vi "u-blox 5 Series Acquire and Chart GPS Advanced.vi"() -> ()   [LabVIEW 2009]
doc: "This example shows how to utilize the advanced VIs in the u-blox 5 GPS driver. It reads the sentences coming from the GPS device and parses out data for position and dilution of precision."
panel:
  out "Dilution of Precision":dbl
  out "Position":cluster{dbl, dbl}[](graph)
  out "Vertical Dilution of Precision":dbl
  out "Horizontal Dilution of Precision":dbl
  in  "stop":bool
  in  "Reset Before Reading (False)":bool
  in  "VISA resource name":refnum<visa-resource-name>
  # "(c) 2009 National Instruments.  ALL RIGHTS RESERVED."
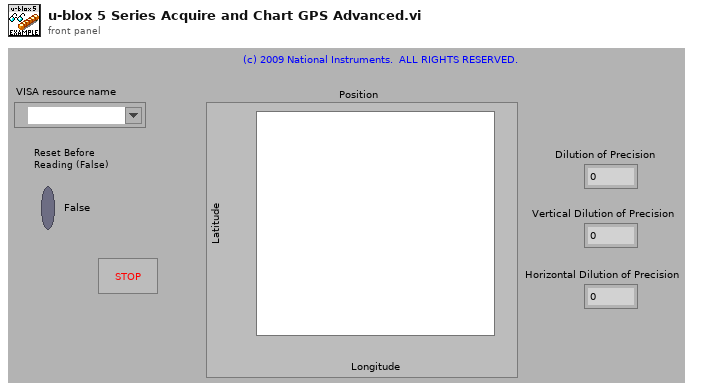
[diagram p1: front panel]
types:
  T1 = cluster{"Dilution of Precision":dbl, "Horizontal Dilution of Precision":dbl, "Vertical Dilution of Precision":dbl}[]
  T2 = cluster{"Timestamp":timestamp, "Latitude":dbl, "Longitude":dbl}[]
  T3 = cluster{"Dilution of Precision":dbl, "Horizontal Dilution of Precision":dbl, "Vertical Dilution of Precision":dbl}
  T4 = cluster{"Timestamp":timestamp, "Latitude":dbl, "Longitude":dbl}
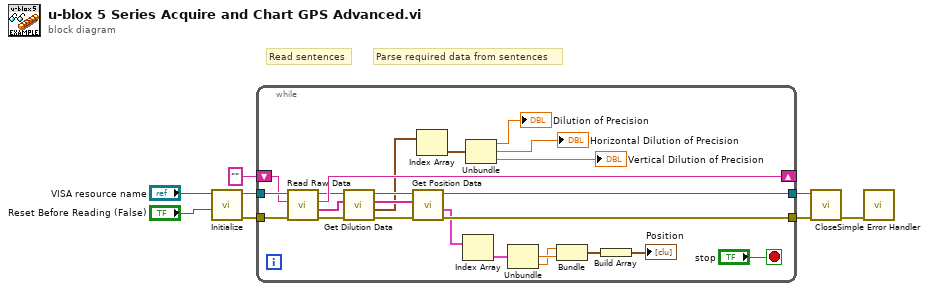
[diagram p0: block diagram]
diagram:
  # "Read sentences"
  # "Parse required data from sentences"
  n1 = call "Initialize.vi"("Reset (False)"="Reset Before Reading (False)", "VISA resource name"="VISA resource name") -> ("error out"=w5:errorcluster, "VISA resource name out"=w6:refnum<visa-resource-name>)  [unwired: 8 in]
  n2 = while {
    tunnel: w6 -> [w32]
    tunnel: w5 -> [w31]
    tunnel: [w22] -> w4
    tunnel: [w21] -> w3
    shift-right: [w29] -> _
    shift-left: "" ("Remaining Partial Sentence") -> [w28]
    stop <- "stop" stop-if-true
    n3 = call "Read Raw Data.vi"("error in (no error)"=w31, "Previous Partial Sentence"=w28, "VISA resource name"=w32) -> ("error out"=w26:errorcluster, "Complete NMEA Sentences"=w17:string[], "Remaining Partial Sentence"=w29:string, "VISA resource name out"=w24:refnum<visa-resource-name>)  [unwired: 5 in]
    n4 = call "Get Dilution Data.vi"("error in (no error)"=w26, "Complete NMEA Sentences"=w17, "VISA resource name"=w24) -> ("error out"=w25:errorcluster, "Dilution Data"=w19:T1, "Complete NMEA Sentences (Copy)"=w20:string[], "VISA resource name out"=w23:refnum<visa-resource-name>)  [unwired: 5 in]
    n5 = call "Get Position Data.vi"("error in (no error)"=w25, "Complete NMEA Sentences"=w20, "VISA resource name"=w23) -> ("error out"=w21:errorcluster, "Position Data"=w18:T2, "VISA resource name out"=w22:refnum<visa-resource-name>)  [unwired: 5 in, 1 out]
    n6 = Index Array(array=w19) -> (element=w16:T3)  [unwired: 1 in]
    n7 = Index Array(array=w18) -> (element=w27:T4)  [unwired: 1 in]
    n8 = Unbundle(w16) -> ("Dilution of Precision"=→"Dilution of Precision":dbl, "Horizontal Dilution of Precision"=→"Horizontal Dilution of Precision":dbl, "Vertical Dilution of Precision"=→"Vertical Dilution of Precision":dbl)
    n9 = Unbundle(w27) -> ("Latitude"=w13:dbl, "Longitude"=w12:dbl)  [unwired: 1 out]
    n10 = Bundle("Longitude"=w12, "Latitude"=w13) -> (w11:cluster{"Longitude":dbl, "Latitude":dbl})  [unwired: 1 in]
    n11 = Build Array(w11) -> (→"Position":cluster{"Longitude":dbl, "Latitude":dbl}[])
  }
  n12 = call "Close.vi"("error in (no error)"=w3, "VISA resource name"=w4) -> ("error out"=w1:errorcluster)  [unwired: 9 in]
  n13 = call <vilib>:"Simple Error Handler.vi"("error in (no error)"=w1) -> ()  [unwired: 4 in, 5 out]
